vi "Read processing parameter.vi"(8 "error in (no error)":errorcluster, 11 "Shared Memory runtime in":refnum<class "Shared Memory runtime.lvclass">) -> (0 "error out":errorcluster, 2 "processing parameter":T4(array[cluster]), 3 "Shared Memory runtime out":refnum<class "Shared Memory runtime.lvclass">)   [LabVIEW 2013, in "Shared Memory runtime.lvclass"]
uses:
  Shared Memory runtime.lvclass
  <vilib>/NI/Tag Bus Module Framework/channel/channel classification.ctl
  <vilib>/NI/Tag Bus/tag/Data Type.ctl
  <vilib>/National Instruments/Shared Memory Library for Linux RT/Controls/Shared Memory Class Reference.ctl
  <vilib>/National Instruments/Shared Memory Library for Linux RT/Classes/Shared Memory/Shared Memory.lvclass
  Shared Memory runtime.lvclass/Shared Memory runtime.ctl
  <vilib>/NI/Tag Bus Module Framework/channel/TBM channel.lvclass
  <vilib>/NI/Tag Bus/tag/tag descriptor.lvclass
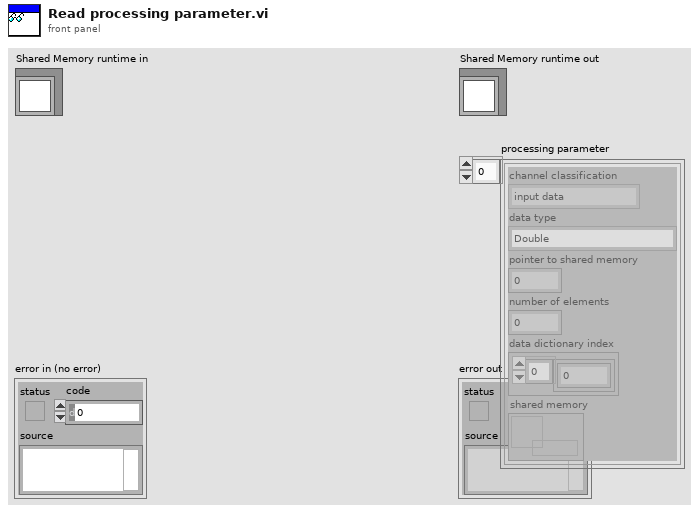
[diagram p1: front panel]
types:
  T1 = typedef "TBM channel.lvclass/channel classification.ctl" = enum16{"input data", "output data", "processing parameter", "processing result"}
  T2 = typedef "tag bus.lvlib/tag descriptor.lvclass/Data Type.ctl" = enum16{"Double", "Single", "I64", "I32", "I16", "I8", "U64", "U32", "U16", "U8", "Boolean", "String", "Array of Double", "Array of Single", "Array of I64", "Array of I32", "Array of I16", "Array of I8", "Array of U64", "Array of U32", "Array of U16", "Array of U8", "Array of Boolean", "Array of String"}
  T3 = typedef "Shared Memory Class Reference.ctl" = refnum<data-value>
  T4 = cluster{"channel classification":T1, "data type":T2, "pointer to shared memory":u64, "number of elements":u64, "data dictionary index":cluster{i32[]}, "shared memory":T3}[]
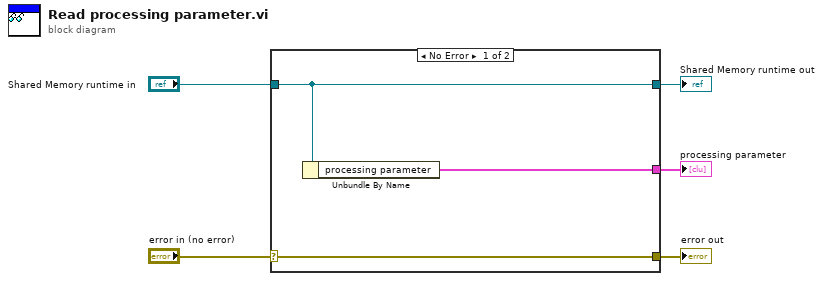
[diagram p0: block diagram]
diagram:
  n1 = case shown="No Error" "error in (no error)" {
    selector: "error in (no error)" -> [w8 w9]
    tunnel: [w8 w9] -> w4
    tunnel: [w7 w10] -> w2
    tunnel: "Shared Memory runtime in" -> [w7 w10]
    tunnel: [w6 _] -> w1
    frame No Error {
      n2 = Unbundle By Name(w7) -> ("processing parameter"=w6:T4)
    }
    frame Error {
    }
  }
  "error out" <- w4
  "Shared Memory runtime out" <- w2
  "processing parameter" <- w1
